vi "ConvetToShow.vi"() -> (4 "远场图":T1, 5 "基本数据":string[](array[string]), 6 "波形":waveform(dbl), 7 "光谱波形":cluster{"X":dbl[], "Y":dbl[]}, 8 "近场图":T1)   [LabVIEW 2018]
uses:
  <vilib>/vision/Image Controls.llb/IMAQ Image.ctl
  Reslut.vi
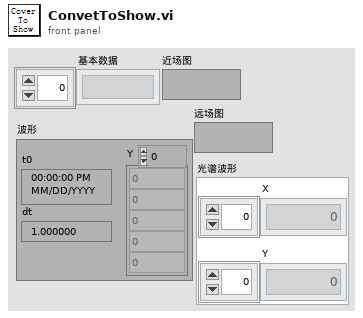
[diagram p1: front panel]
types:
  T1 = typedef "IMAQ Image.ctl" = refnum<image>
  T2 = cluster{"近场图":T1, " 远场图":T1, "发散角X/rad":dbl, "发散角Y/rad":dbl, "近场图 buffer":T1, "发散角采集完成":bool}
  T3 = cluster{"波形":waveform(dbl), "脉宽":string, "重频":string, "脉冲宽度Uint":string, "重复频率Uint":string}
  T4 = cluster{"能量计结果":string, "功率计结果":string, "能量计单位":string, " 功率计单位":string}
  T5 = cluster{"光谱波形":cluster{"X":dbl[], "Y":dbl[]}, "中心波长":string, " 谱宽":string, " 中心波长Uint":string, " 谱宽 Uint":string}
  T6 = cluster{" 偏振方向":string, "偏振度":string, " 偏振方向 单位 ":string, "偏振度单位":string}
  T7 = cluster{"激光器型号":string, "X":dbl, "Y":dbl, "Z":dbl, "Rotate":dbl, "Pitching":dbl, "DivergeAngle":dbl}
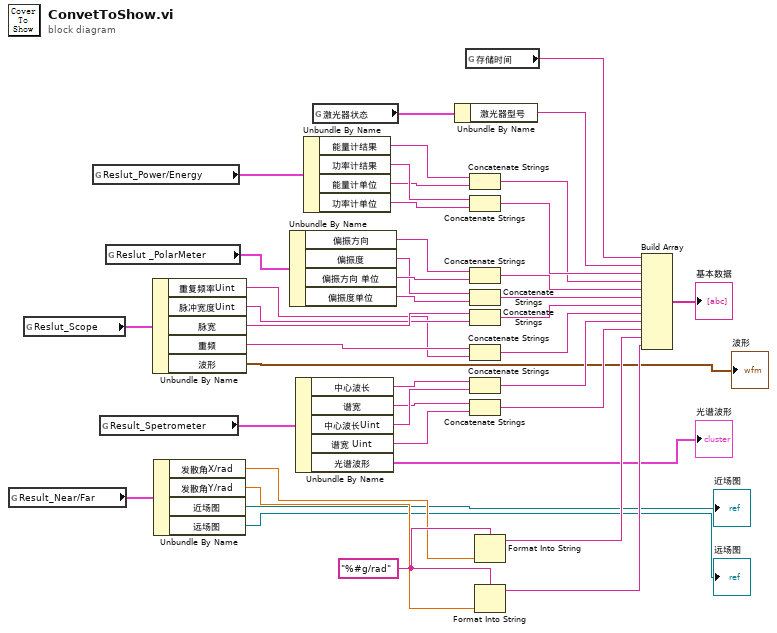
[diagram p0: block diagram]
diagram:
  w10 = "%#g/rad" ("格式字符串")
  n1 = global read "Reslut.vi" "Result_Near/Far"() -> (w11:T2)
  n2 = global read "Reslut.vi" "Reslut_Scope"() -> (w25:T3)
  n3 = global read "Reslut.vi" "Reslut_Power/Energy"() -> (w42:T4)
  n4 = global read "Reslut.vi" "Result_Spetrometer"() -> (w18:T5)
  n5 = global read "Reslut.vi" "Reslut _PolarMeter"() -> (w32:T6)
  n6 = Unbundle By Name(w25) -> ("重复频率Uint"=w21:string, "脉冲宽度Uint"=w23:string, "脉宽"=w24:string, "重频"=w22:string, "波形"=→"波形":waveform(dbl))
  n7 = Unbundle By Name(w11) -> ("发散角X/rad"=w9:dbl, "发散角Y/rad"=w8:dbl, "近场图"=→"近场图":T1, "远场图"=→"远场图":T1)
  n8 = Unbundle By Name(w32) -> ("偏振方向"=w31:string, "偏振度"=w29:string, "偏振方向 单位"=w30:string, "偏振度单位"=w28:string)
  n9 = Unbundle By Name(w18) -> ("中心波长"=w17:string, "谱宽"=w15:string, "中心波长Uint"=w16:string, "谱宽 Uint"=w14:string, "光谱波形"=→"光谱波形":cluster{"X":dbl[], "Y":dbl[]})
  n10 = Unbundle By Name(w42) -> ("能量计结果"=w39:string, "功率计结果"=w41:string, "能量计单位"=w38:string, "功率计单位"=w40:string)
  n11 = global read "参数.vi" "激光器状态"() -> (w34:T7)
  n12 = Unbundle By Name(w34) -> ("激光器型号"=w33:string)
  n13 = global read "Reslut.vi" "存储时间"() -> (w35:string)
  n14 = Concatenate Strings(w39, w38) -> (w36:string)
  n15 = Concatenate Strings(w41, w40) -> (w37:string)
  n16 = Concatenate Strings(w31, w30) -> (w27:string)
  n17 = Concatenate Strings(w29, w28) -> (w26:string)
  n18 = Concatenate Strings(w24, w23) -> (w20:string)
  n19 = Concatenate Strings(w22, w21) -> (w19:string)
  n20 = Concatenate Strings(w17, w16) -> (w13:string)
  n21 = Concatenate Strings(w15, w14) -> (w12:string)
  n22 = Format Into String(format string=w10, w9) -> (resulting string=w7:string)  [unwired: 2 in, 1 out]
  n23 = Format Into String(format string=w10, w8) -> (resulting string=w6:string)  [unwired: 2 in, 1 out]
  n24 = Build Array(w35, w33, w37, w36, w27, w26, w20, w19, w13, w12, w7, w6) -> (→"基本数据":string[])
